vi "SVL Unit Conversion (XY) (1 Ch).vi"(0 "magnitudes":cluster{"time/rev/rpm":dbl[], "magnitude":dbl[]} {"magnitude" format="%.2f"; "time/rev/rpm" format="%.2f"}, 1 "desired scaling":T1 {"dB reference (0: no change)" format="%.2f"}, 4 "magnitude info in":T2={"channel name"="", "description"="", "x-axis units"=0, "spectral info"={"spectrum type"=enum."Power [Magnitude^2]", "linear/dB"=enum."linear", "window"=0, "window size"=0, "FFT size"=0}, "engineering units"=0, "custom label"="", "dB reference [EU]"=0.0, "peak units"=enum."rms", "weighting filter"=0, "spectral density?"=FALSE, "unit label"="", "spectrum skewed?"=FALSE, "complimentary spectrum units"=enum."none"} {"x-axis units" items=["Time (s)"=0, "Frequency-CB (Hz)"=1, "Frequency-CPB (Hz)"=1248, "Frequency-Arbitrary (Hz)"=2357, "Quefrency (s)"=2, "Revolutions (rev)"=3, "Order"=4, "Speed (RPM)"=11, "Speed (rad/s)"=21, "Index"=65535]; "weighting filter" items=["Linear", "A-weighting", "B-weighting", "C-weighting", "ITU-R 468-4", "Dolby", "CCITT", "C-message", "Wb", "Wc", "Wd", "We", "Wf", "Wh", "Wj", "Wk", "Wm", "AES17 20 kHz lowpass", "AES17 40 kHz lowpass", "AES17 20 kHz highpass", "AES17 40 kHz highpass"]; "dB reference [EU]" format="%.2f"; "engineering units" items=["custom..."=0, "V"=1, "A"=21, "C"=30, "pC"=31, "s"=32, "-"=29, "Pa"=2, "N"=20, "g"=3, "m/s^2"=4, "m/s"=5, "m"=6, "mm/s"=12, "mm"=13, "micron/s"=14, "micron"=15, "in/s^2"=7, "in/s"=8, "in"=9, "mil/s"=10, "mil"=11, "rad/s^2"=16, "rad/s"=17, "rad"=18, "deg/s^2"=26, "deg/s"=27, "deg"=28, "RPM"=22, "cycle/s^2"=23, "Hz"=24, "cycle"=25, "strain"=19]; "spectral info"."window" items=["None "=0, "Hanning"=1, "Hamming"=2, "Blackman-Harris"=3, "Exact Blackman"=4, "Blackman"=5, "Flat Top"=6, "4 Term B-Harris "=7, "7 Term B-Harris"=8, "Low Sidelobe"=9, "Force - Exponential"=10, "Gaussian"=62]}, 5 "error in (no error)":errorcluster) -> (14 "converted magnitudes":cluster{"time/rev/rpm":dbl[], "magnitude":dbl[]} {"magnitude" format="%.2f"; "time/rev/rpm" format="%.2f"}, 15 "unit label":string, 18 "magnitude info out":T2={"channel name"="", "description"="", "x-axis units"=0, "spectral info"={"spectrum type"=enum."Power [Magnitude^2]", "linear/dB"=enum."linear", "window"=0, "window size"=0, "FFT size"=0}, "engineering units"=0, "custom label"="", "dB reference [EU]"=0.0, "peak units"=enum."rms", "weighting filter"=0, "spectral density?"=FALSE, "unit label"="", "spectrum skewed?"=FALSE, "complimentary spectrum units"=enum."none"} {"x-axis units" items=["Time (s)"=0, "Frequency-CB (Hz)"=1, "Frequency-CPB (Hz)"=1248, "Frequency-Arbitrary (Hz)"=2357, "Quefrency (s)"=2, "Revolutions (rev)"=3, "Order"=4, "Speed (RPM)"=11, "Speed (rad/s)"=21, "Index"=65535]; "weighting filter" items=["Linear", "A-weighting", "B-weighting", "C-weighting", "ITU-R 468-4", "Dolby", "CCITT", "C-message", "Wb", "Wc", "Wd", "We", "Wf", "Wh", "Wj", "Wk", "Wm", "AES17 20 kHz lowpass", "AES17 40 kHz lowpass", "AES17 20 kHz highpass", "AES17 40 kHz highpass"]; "dB reference [EU]" format="%.2f"; "engineering units" items=["custom..."=0, "V"=1, "A"=21, "C"=30, "pC"=31, "s"=32, "-"=29, "Pa"=2, "N"=20, "g"=3, "m/s^2"=4, "m/s"=5, "m"=6, "mm/s"=12, "mm"=13, "micron/s"=14, "micron"=15, "in/s^2"=7, "in/s"=8, "in"=9, "mil/s"=10, "mil"=11, "rad/s^2"=16, "rad/s"=17, "rad"=18, "deg/s^2"=26, "deg/s"=27, "deg"=28, "RPM"=22, "cycle/s^2"=23, "Hz"=24, "cycle"=25, "strain"=19]; "spectral info"."window" items=["None "=0, "Hanning"=1, "Hamming"=2, "Blackman-Harris"=3, "Exact Blackman"=4, "Blackman"=5, "Flat Top"=6, "4 Term B-Harris "=7, "7 Term B-Harris"=8, "Low Sidelobe"=9, "Force - Exponential"=10, "Gaussian"=62]}, 19 "error out":errorcluster)   [LabVIEW 2017]
doc: "Converts between dB/linear, magnitude/magnitude^2, rms/peak/peak-peak, spectrum/spectral density, and dB ref1/dB ref2. You can use this polymorphic VI to convert a single spectrum, N spectra, a single complex spectrum, N complex spectra, a single channel of XY data, N channels of XY data, a single channel with M orders of XY data, N channels with M orders of XY data, waterfall data, or colormap data. The data type you wire to the <B>spectrum</B> or <B>magnitudes</B> input determines the polymorphic instance to use."
uses:
  <vilib>/addons/_NISVFA/_Shared subVIs/Controls/svc_Spectrum Info.ctl
  <vilib>/addons/_NISVFA/_Shared subVIs/Controls/svc_X-Axis Units.ctl
  <vilib>/addons/_NISVFA/_Shared subVIs/Controls/svc_Spectrum Type.ctl
  <vilib>/addons/_NISVFA/_Shared subVIs/Controls/svc_Engineering Units Text Ring.ctl
  <vilib>/addons/_NISVFA/_Shared subVIs/Controls/svc_Weighting Filter Text Ring.ctl
  <vilib>/addons/_NISVFA/_Shared subVIs/Controls/svc_Complimentary Spectrum Units.ctl
  <vilib>/addons/_NISVFA/_Spectrum Processing/subVIs/svfa_Peak to RMS to Peak2Peak.vi
  <vilib>/addons/_NISVFA/_Spectrum Processing/subVIs/svfa_Mag to Mag2.vi
  <vilib>/addons/_NISVFA/_Spectrum Processing/subVIs/svfa_Linear to dB.vi
  <vilib>/addons/_NISVFA/_Spectrum Processing/subVIs/svfa_dBrefA to dBrefB.vi
  <vilib>/addons/_NISVFA/_Spectrum Processing/subVIs/svfa_Spectrum to Spectral Density.vi
  <vilib>/addons/_NISVFA/_Shared subVIs/Common/svc_Get Weighting Enum and Labels.vi
  <vilib>/addons/_NISVFA/_Shared subVIs/Common/svc_Unit Label Lexical Class.vi
  <vilib>/addons/_NISVFA/_Shared subVIs/Common/svc_Engineering Units to Unit Label.vi
  <vilib>/addons/_NISVFA/_Shared subVIs/Common/svc_Format Value (DBL).vi
  <vilib>/addons/_NISVFA/_Shared subVIs/Common/svc_Window Parameters.vi
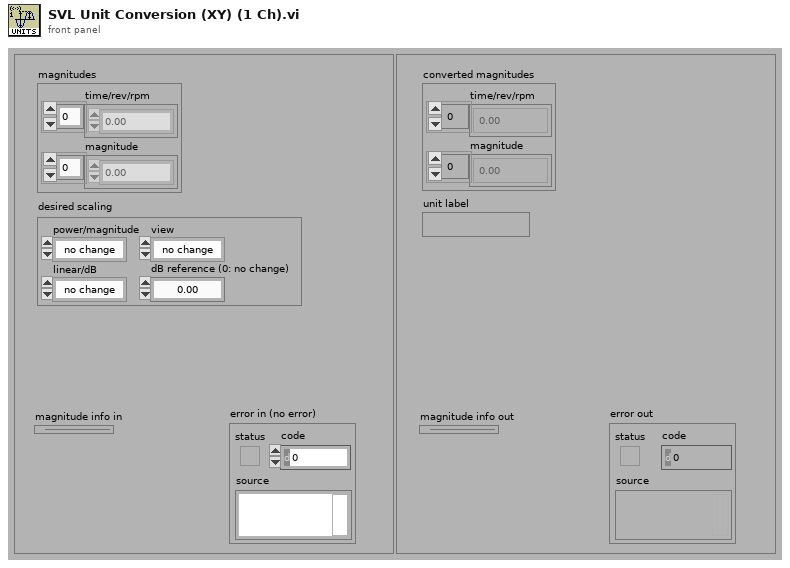
[diagram p1: front panel]
types:
  T1 = cluster{"linear/dB":enum16{"no change", "linear", "dB"}, "dB reference (0: no change)":dbl, "power/magnitude":enum16{"no change", "power", "magnitude"}, "view":enum16{"no change", "rms", "peak", "peak-peak"}}
  T2 = typedef "svc_Spectrum Info.ctl" = cluster{"channel name":string, "description":string, "x-axis units":T3, "spectral info":cluster{"spectrum type":T4, "linear/dB":enum16{"linear", "dB"}, "window":u16, "window size":i32, "FFT size":i32}, "engineering units":T5, "custom label":string, "dB reference [EU]":dbl, "peak units":enum16{"rms", "peak", "peak-peak"}, "weighting filter":T6, "spectral density?":bool, "unit label":string, "spectrum skewed?":bool, "complimentary spectrum units":T7}
  T3 = typedef "svc_X-Axis Units.ctl" = u16
  T4 = typedef "svc_Spectrum Type.ctl" = enum16{"FFT Spectrum [complex]", "Amplitude [Magnitude]", "Power [Magnitude^2]", "Cross Spectrum [complex]", "Frequency Response [Complex]"}
  T5 = typedef "svc_Engineering Units Text Ring.ctl" = u16
  T6 = typedef "svc_Weighting Filter Text Ring.ctl" = u16
  T7 = typedef "svc_Complimentary Spectrum Units.ctl" = enum16{"none", "radians", "degrees", "cycles", "imaginary"}
  T8 = enum16{"no change", "spectrum", "spectral density"}
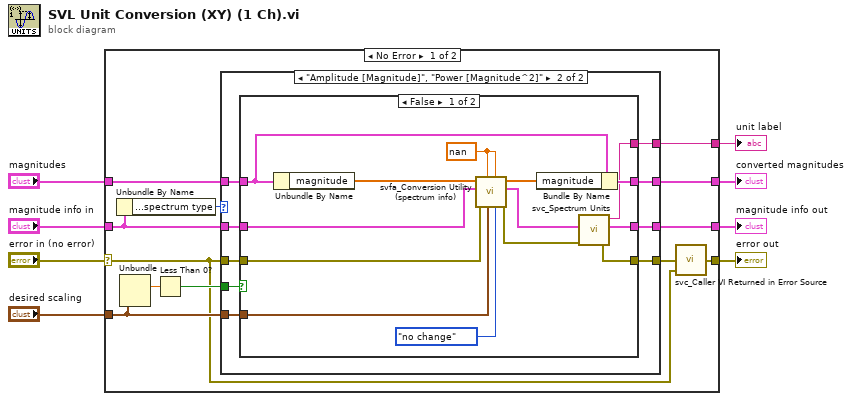
[diagram p0: block diagram]
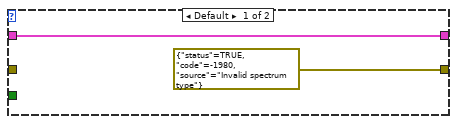
[diagram p2: hidden frame]
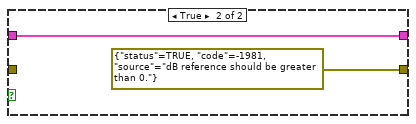
[diagram p3: hidden frame]
diagram:
  n1 = case shown="No Error" "error in (no error)" {
    selector: "error in (no error)" -> [w9 w50]
    tunnel: [w15 w50] -> w7
    tunnel: "magnitudes" -> [w20 w48]
    tunnel: "desired scaling" -> [w12 _]
    tunnel: [w19 w48] -> w5
    tunnel: "magnitude info in" -> [w14 w49]
    tunnel: [w16 w49] -> w2
    tunnel: [w17 _] -> w1
    frame No Error {
      n2 = Unbundle By Name(w14) -> ("spectral info.spectrum type"=w13:T4)
      n3 = Unbundle(w12) -> ("dB reference (0: no change)"=w11:dbl)  [unwired: 3 out]
      n4 = Less Than 0?(x=w11) -> (x < 0?=w10:bool)
      n5 = case shown="\"Amplitude [Magnitude]\", \"Power [Magnitude^2]\"" w13 {
        tunnel: w20 -> [_ w31]
        tunnel: [_ w30] -> w19
        tunnel: w9 -> [_ w29]
        tunnel: w12 -> [_ w28]
        tunnel: [errorcluster {"status"=TRUE, "code"=-1980, "source"="Invalid spectrum type"} ("error out") w27] -> w18
        tunnel: [_ w26] -> w17
        tunnel: [w21 w25] -> w16
        tunnel: w14 -> [w21 w24]
        tunnel: w10 -> [_ w23]
        frame Default {
        }
        frame "Amplitude [Magnitude]", "Power [Magnitude^2]" {
          n6 = case shown="False" w23 {
            tunnel: w31 -> [w45 _]
            tunnel: [w44 _] -> w30
            tunnel: w29 -> [w40 _]
            tunnel: w28 -> [w43 _]
            tunnel: [w35 errorcluster {"status"=TRUE, "code"=-1981, "source"="dB reference should be greater than 0."} ("error out")] -> w27
            tunnel: [w34 _] -> w26
            tunnel: [w36 w47] -> w25
            tunnel: w24 -> [w38 w47]
            frame False {
              w32 = nan ("dx")
              n7 = Unbundle By Name(w45) -> ("magnitude"=w41:dbl[])
              n8 = call <vilib>:"svfa_Conversion Utility (spectrum info).vi"("spectral density desired"=T8."no change", "dx"=w32, "desired scaling"=w43, "x0"=w32, "error in (no error)"=w40, "spectrum info in"=w38, "input signal"=w41) -> ("error out"=w39:errorcluster, "spectrum info out"=w37:T2, "converted signal"=w42:dbl[])  [unwired: 2 in]
              n9 = Bundle By Name(cluster=w45, "magnitude"=w42) -> (w44:cluster{"time/rev/rpm":dbl[], "magnitude":dbl[]})
              n10 = call <vilib>:"svc_Spectrum Units.vi"("error in (no error)"=w39, "spectrum info in"=w37) -> ("error out"=w35:errorcluster, "spectrum info out"=w36:T2, "unit label"=w34:string)  [unwired: 2 in, 1 out]
            }
            frame True {
            }
          }
        }
      }
      n11 = call <vilib>:"svc_Caller VI Returned in Error Source.vi"("warning input to caller"=w9, "error in (no error)"=w18) -> ("error out"=w15:errorcluster)  [unwired: 3 in]
    }
    frame Error {
    }
  }
  "error out" <- w7
  "converted magnitudes" <- w5
  "magnitude info out" <- w2
  "unit label" <- w1
